vi "Projection.vi"(10 "Axis":T1, 11 "Hailstone in":refnum<class "Vector.lvclass">) -> (2 "Trace":refnum<class "Trace.lvclass">)   [LabVIEW 2021]
uses:
  Vector.lvclass
  Trace/Trace.lvclass
  Proto/Plane.ctl
  Vector.lvclass/Vector.ctl
  High Res Arithmetic/High Res Arithmetic.lvclass
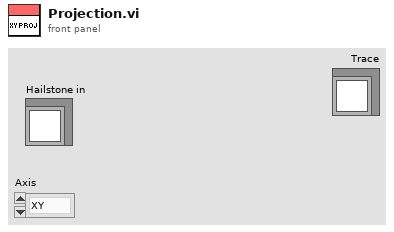
[diagram p1: front panel]
types:
  T1 = typedef "Plane.ctl" = enum16{"XY", "YX"}
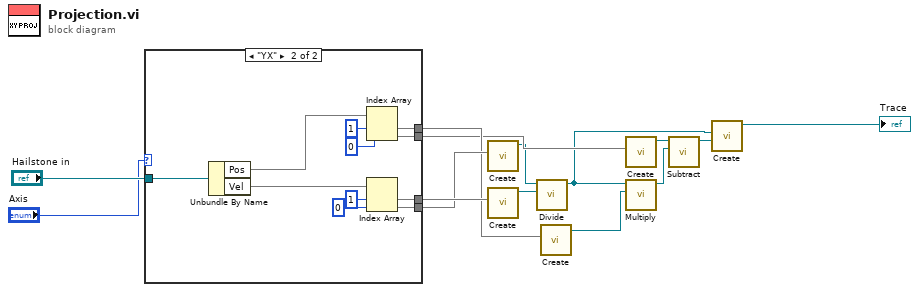
[diagram p0: block diagram]
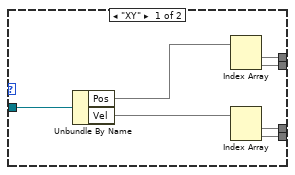
[diagram p2: hidden frame]
diagram:
  n1 = case shown="\"YX\"" "Axis" {
    tunnel: "Hailstone in" -> [w20 w31]
    tunnel: [w18 w29] -> w12
    tunnel: [w17 w28] -> w11
    tunnel: [w16 w27] -> w9
    tunnel: [w15 w26] -> w7
    frame "XY" {
      n2 = Unbundle By Name(w20) -> ("Pos"=w21, "Vel"=w19)
      n3 = Index Array(array=w21) -> (element #1=w16, element #2=w15)  [unwired: 2 in]
      n4 = Index Array(array=w19) -> (element #1=w18, element #2=w17)  [unwired: 2 in]
    }
    frame "YX" {
      n5 = Unbundle By Name(w31) -> ("Pos"=w32, "Vel"=w30)
      n6 = Index Array(array=w32, index #1=1 ("index"), index #2=0 ("index")) -> (element #1=w27, element #2=w26)
      n7 = Index Array(array=w30, index #1=1 ("index"), index #2=0 ("index")) -> (element #1=w29, element #2=w28)
    }
  }
  n8 = call "Create.vi"("Numerator"=w11) -> ("Hi Res Arithm Test"=w3:refnum<class "High Res Arithmetic.lvclass">)  [unwired: 9 in, 1 out]
  n9 = call "Create.vi"("Numerator"=w12) -> ("Hi Res Arithm Test"=w10:refnum<class "High Res Arithmetic.lvclass">)  [unwired: 9 in, 1 out]
  n10 = call "Divide.vi"("High Res Arithmetic 2"=w10, "High Res Arithmetic 1"=w3) -> ("High Res Arithmetic sum"=w2:refnum<class "High Res Arithmetic.lvclass">)  [unwired: 8 in, 1 out]
  n11 = call "Create.vi"("Numerator"=w9) -> ("Hi Res Arithm Test"=w8:refnum<class "High Res Arithmetic.lvclass">)  [unwired: 9 in, 1 out]
  n12 = call "Create.vi"("Numerator"=w7) -> ("Hi Res Arithm Test"=w6:refnum<class "High Res Arithmetic.lvclass">)  [unwired: 9 in, 1 out]
  n13 = call "Multiply.vi"("High Res Arithmetic 2"=w8, "High Res Arithmetic 1"=w2) -> ("High Res Arithmetic sum"=w5:refnum<class "High Res Arithmetic.lvclass">)  [unwired: 8 in, 1 out]
  n14 = call "Subtract.vi"("High Res Arithmetic 2"=w5, "High Res Arithmetic 1"=w6) -> ("High Res Arithmetic sum"=w4:refnum<class "High Res Arithmetic.lvclass">)  [unwired: 8 in, 1 out]
  n15 = call "Create.vi"("Offset"=w4, "Slope"=w2) -> ("Trace"=→"Trace":refnum<class "Trace.lvclass">)  [unwired: 8 in, 1 out]
